vi "Check Re-Arm Ticks Done.vi"(8 "Increment?":bool, 9 "Re-Arm Ticks":u16, 11 "Re-Arm Ticks to Wait":u16) -> (1 "Updated Re-Arm Ticks":u16, 3 "Re-Arm Ticks Done?":bool)   [LabVIEW 2012]
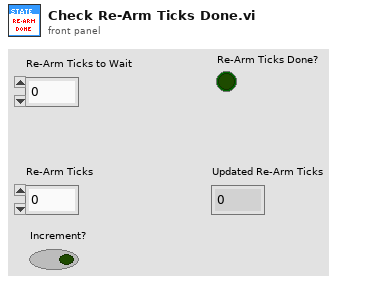
[diagram p1: front panel]
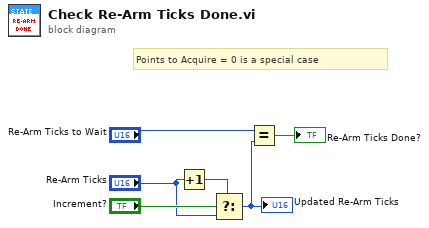
[diagram p0: block diagram]
diagram:
  # "Points to Acquire = 0 is a special case"
  n1 = Increment(x="Re-Arm Ticks") -> (x+1=w6:u16)
  n2 = Select(t=w6, s="Increment?", f="Re-Arm Ticks") -> (s? t:f=w3:u16)
  "Updated Re-Arm Ticks" <- w3
  n3 = Equal?(x="Re-Arm Ticks to Wait", y=w3) -> (x = y?=→"Re-Arm Ticks Done?":bool)
